vi "Set DDS Sweep Time.vi"(10 "time_ns":cluster{}, 11 "channel_index":u8) -> ()   [LabVIEW 2021, in "vmmso.lvlib"]
doc: "DLL_API void WINAPI SetDDSSweepTime(unsigned char channel_index, unsigned long long int time_ns);"
uses:
  vmmso.lvlib
  vmmso.dll
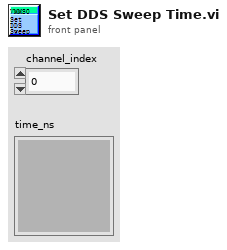
[diagram p1: front panel]
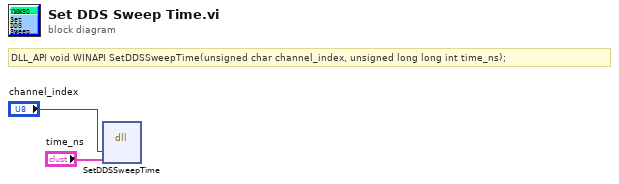
[diagram p0: block diagram]
diagram:
  # "DLL_API void WINAPI SetDDSSweepTime(unsigned char channel_index, unsigned long long int time_ns);"
  n1 = dll-call lib="D:/labviewdemo/LabviewDemo 21/vmmso/vmmso.*" fn="SetDDSSweepTime"("channel_index"="channel_index", "time_ns"="time_ns") -> ()  [unwired: 6 in, 2 out]
